vi "SavePosition_KCubeInertial.vi"(4 "start/stop write":bool, 5 "init file":bool, 7 "Device":refnum<k24>, 8 "state in":T1(ring), 9 "filename save":string, 10 "Folder path save":path, 11 "Byte Stream File in":refnum<file>) -> (0 "state out":T1(ring), 2 "current state":string, 3 "Byte Stream File out":refnum<file>)   [LabVIEW 2019]
doc: "saves datetime, position value, and ischannelbusy for channel 1 of inertial motor"
uses:
  D:/Victor Sun/optical trap control/Kinesis/Thorlabs.MotionControl.KCube.InertialMotorCLI.dll
  Kinesis/Thorlabs.MotionControl.KCube.InertialMotorCLI.dll
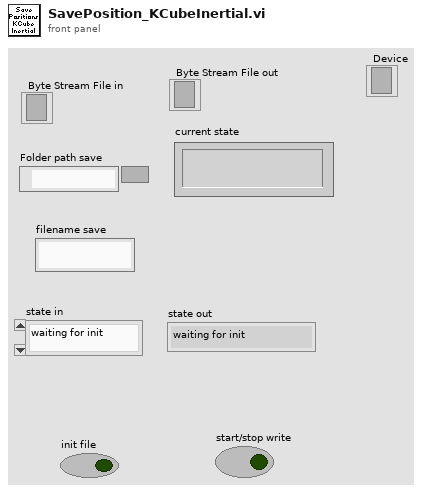
[diagram p1: front panel]
types:
  T1 = enum16{"waiting for init", "init", "waiting for write", "write", "stop", ""}
  T2 = enum16{"open", "replace", "create", "open or create", "replace or create", "replace or create with confirmation"}
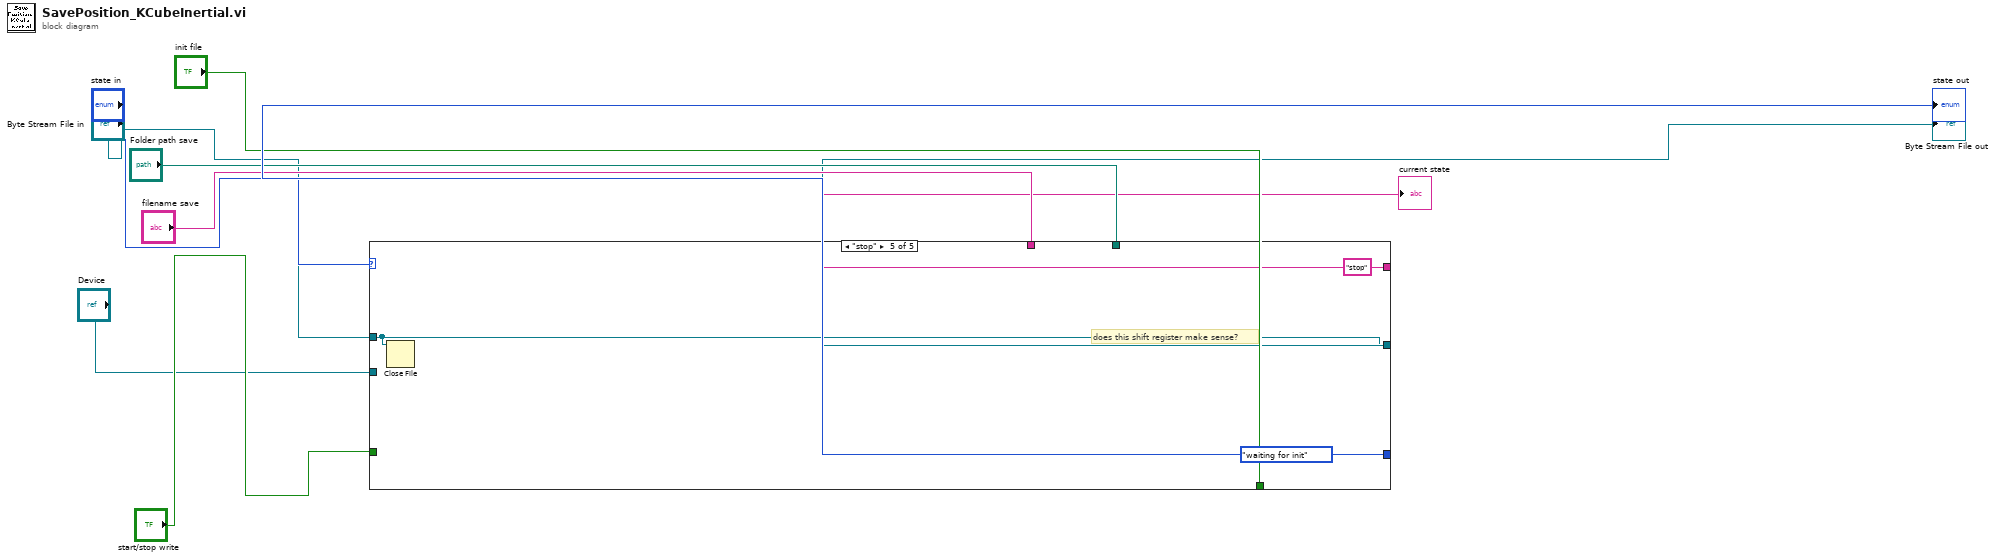
[diagram p0: block diagram]
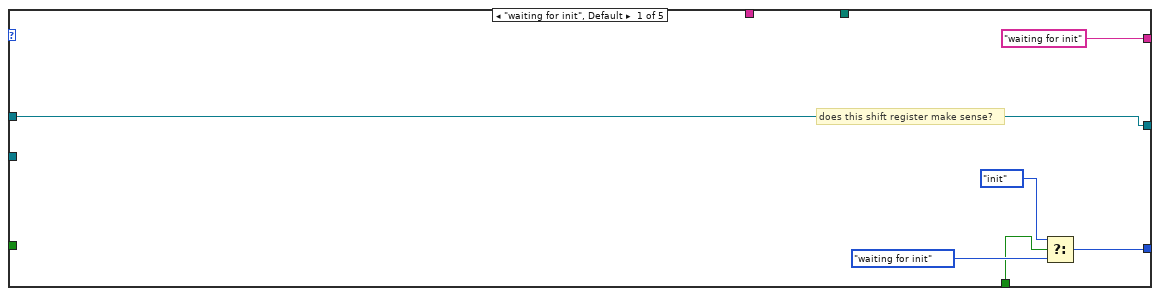
[diagram p2: hidden frame]
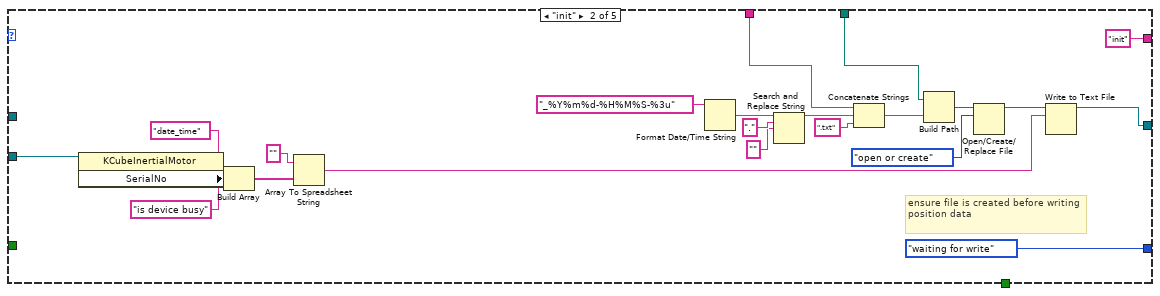
[diagram p3: hidden frame]
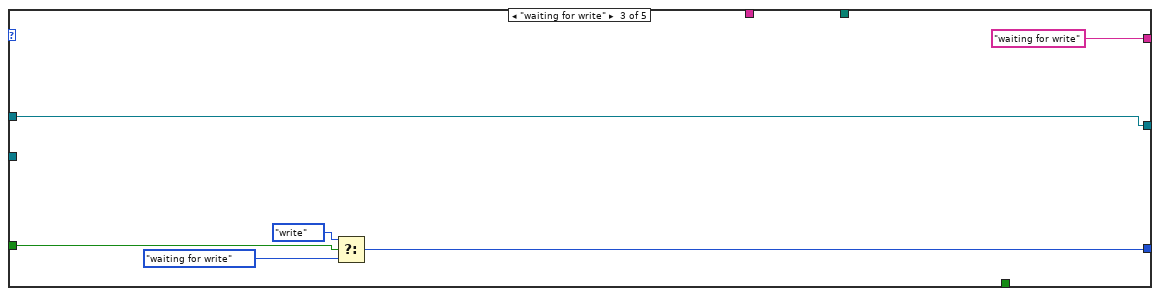
[diagram p4: hidden frame]
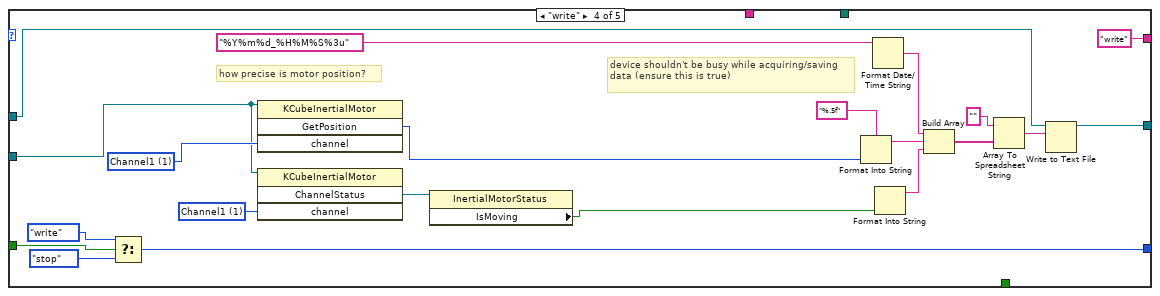
[diagram p5: hidden frame]
diagram:
  n1 = case shown="\"stop\"" "state in" {
    tunnel: [w15 T1."waiting for write" w43 w64 T1."waiting for init"] -> w10
    tunnel: ["waiting for init" ("String") "init" ("String") "waiting for write" ("String") "write" ("String") "stop" ("String")] -> w1
    tunnel: "Device" -> [_ w20 _ w46 _]
    tunnel: [w11 w19 w40 w62 w66] -> w3
    tunnel: "Byte Stream File in" -> [w11 _ w40 w63 w66]
    tunnel: "start/stop write" -> [_ _ w39 w53 _]
    tunnel: "init file" -> [w13 _ _ _ _]
    tunnel: "filename save" -> [_ w32 _ _ _]
    tunnel: "Folder path save" -> [_ w29 _ _ _]
    frame "waiting for init", Default {
      # "does this shift register make sense?"
      n2 = Select(t=T1."init", s=w13, f=T1."waiting for init") -> (s? t:f=w15:T1)
    }
    frame "init" {
      # "ensure file is created before writing position data"
      n3 = property class="KCubeInertialMotor"(reference=w20) -> ("SerialNo"=w22:string)  [unwired: 1 in, 2 out]
      n4 = Build Array("date_time", w22, "is device busy" ("element")) -> (w21:string[])
      n5 = Array To Spreadsheet String(array=w21, 3:"" ("format string")) -> (spreadsheet string=w35:string)  [unwired: 1 in]
      n6 = Format Date/Time String(time format string (%c)="_%Y%m%d-%H%M%S-%3u") -> (date/time string=w30:string)  [unwired: 2 in]
      n7 = Search and Replace String(input string=w30, search string=".", replace string="" ("replace string (\"\")")) -> (result string=w31:string)  [unwired: 5 in, 3 out]
      n8 = Concatenate Strings(w32, w31, ".txt" ("result string")) -> (w33:string)
      n9 = Build Path(base path=w29, name or relative path=w33) -> (appended path=w34:path)
      n10 = Open/Create/Replace File(file path (use dialog)=w34, operation (0:open)=T2."open or create") -> (refnum out=w36:refnum<file>)  [unwired: 4 in, 2 out]
      n11 = Write to Text File(file (use dialog)=w36, text=w35) -> (refnum out=w19:refnum<file>)  [unwired: 2 in, 2 out]
    }
    frame "waiting for write" {
      n12 = Select(t=T1."write", s=w39, f=T1."waiting for write") -> (s? t:f=w43:T1)
    }
    frame "write" {
      w49 = 1 items=["Channel1"=1, "Channel2"=2, "Channel3"=3, "Channel4"=4] ("channel")
      w48 = 1 items=["Channel1"=1, "Channel2"=2, "Channel3"=3, "Channel4"=4] ("channel")
      # "device shouldn't be busy while acquiring/saving data (ensure this is true)"
      # "how precise is motor position?"
      n13 = Select(t=T1."write", s=w53, f=T1."stop") -> (s? t:f=w64:T1)
      n14 = invoke class="KCubeInertialMotor" method="GetPosition"(reference=w46, "channel"=w48) -> ("GetPosition"=w45:i32)  [unwired: 2 in, 3 out]
      n15 = invoke class="KCubeInertialMotor" method="ChannelStatus"(reference=w46, "channel"=w49) -> ("ChannelStatus"=w50:refnum<k24>)  [unwired: 2 in, 3 out]
      n16 = property class="InertialMotorStatus"(reference=w50) -> ("IsMoving"=w47:bool)  [unwired: 1 in, 2 out]
      n17 = Format Into String(format string="%.5f", w45) -> (resulting string=w58:string)  [unwired: 2 in, 1 out]
      n18 = Format Date/Time String(time format string (%c)="%Y%m%d_%H%M%S%3u") -> (date/time string=w59:string)  [unwired: 2 in]
      n19 = Format Into String(w47) -> (resulting string=w54:string)  [unwired: 3 in, 1 out]
      n20 = Build Array(w59, w58, w54) -> (w57:string[])
      n21 = Array To Spreadsheet String(array=w57, 3:"" ("format string")) -> (spreadsheet string=w56:string)  [unwired: 1 in]
      n22 = Write to Text File(file (use dialog)=w63, text=w56) -> (refnum out=w62:refnum<file>)  [unwired: 2 in, 2 out]
    }
    frame "stop" {
      # "does this shift register make sense?"
      n23 = Close File(refnum=w66) -> ()  [unwired: 1 in, 2 out]
    }
  }
  "current state" <- w1
  "state out" <- w10
  "Byte Stream File out" <- w3
